vi "OM State Strings 2 Messages.vi"() -> (1 "OM State Strings":T1, 3 "Messages":string)   [LabVIEW 2009]
uses:
  OM State Strings.ctl
  App Status Actions.ctl
  Data Access Objects/Metadata/Persistant DAO Actions.ctl
  Lbcb Control Loop States.ctl
  Data Access Objects/Application/Number Of LBCBs.ctl
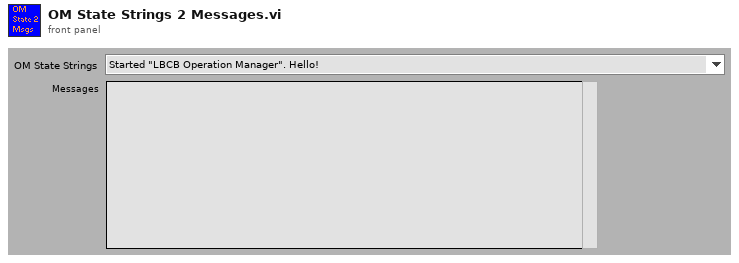
[diagram p1: front panel]
types:
  T1 = typedef "OM State Strings.ctl" = enum16{"Started \"LBCB Operation Manager\". Hello!", "Loading Configuration...", "Setting Up Archiving ...", "Setting Up DAQ Channels...", "Starting Data Acquisition....", "Examine Command from last run ...", "Running  Auto-Balance feedback control loop for LBCB 1 ...", "Running  Auto-Balance feedback control loop for LBCB 2 ...", "Ready to start \"Control\" process for LBCB 1. Push \"Control\" button. ", "Ready to start \"Control\" process for LBCB 2. Push \"Control\" button. ", "LBCB 1 under control", "LBCB 2 under control", "Starting control process. Ready to turn on the pump!", "Stopped \"LBCB Operation Manager\". Bye!"}
  T2 = typedef "Number Of LBCBs.ctl" = enum16{"1", "2"}
  T3 = typedef "Lbcb Control Loop States.ctl" = enum16{"Idle", "Load Last Command", "Start Autobalancing", "Autobalancing", "Control Loop Initialized", "Control Enabled"}
  T4 = typedef "Persistant DAO Actions.ctl" = enum16{"Init", "Get", "Set", "Load", "Save"}
  T5 = typedef "App Status Actions.ctl" = enum16{"Init", "Get Status", "Running", "Control", "Autobalanced", "Data Acquisition", "Set App State", "DAQ Started", "Set LBCB State", "Set All", "Set Cont Logging", "Set Step Logging", "Set MM Logging", "Set Volt Logging", "Set Cart Type", "Set DAQ Link"}
  T6 = typedef "App Status.ctl" = cluster{"Running":bool, "Controlling L2":bool, "Autobalance L2":bool, "Data Acquisition":bool, " App State":T7, "DAQ Started":bool, "LBCB 1 State":T3, "LBCB 2 State":T3, "Controlling L1":bool, "Autobalance L1":bool, "Cartesian Type":bool, "Continuous Logging":bool, "Step Logging":bool, "Voltage Logging":bool, "Mixed Mode Logging":bool, "DAQ Link":bool}
  T7 = typedef "AppStates.ctl" = enum16{"Starting OM", "Initializing Displays", "Setting up Archiving", "Setting Up DAQ Channels", "Start DAQ", "DAQ Starting", "Controlling LBCBs", "Stopping OM"}
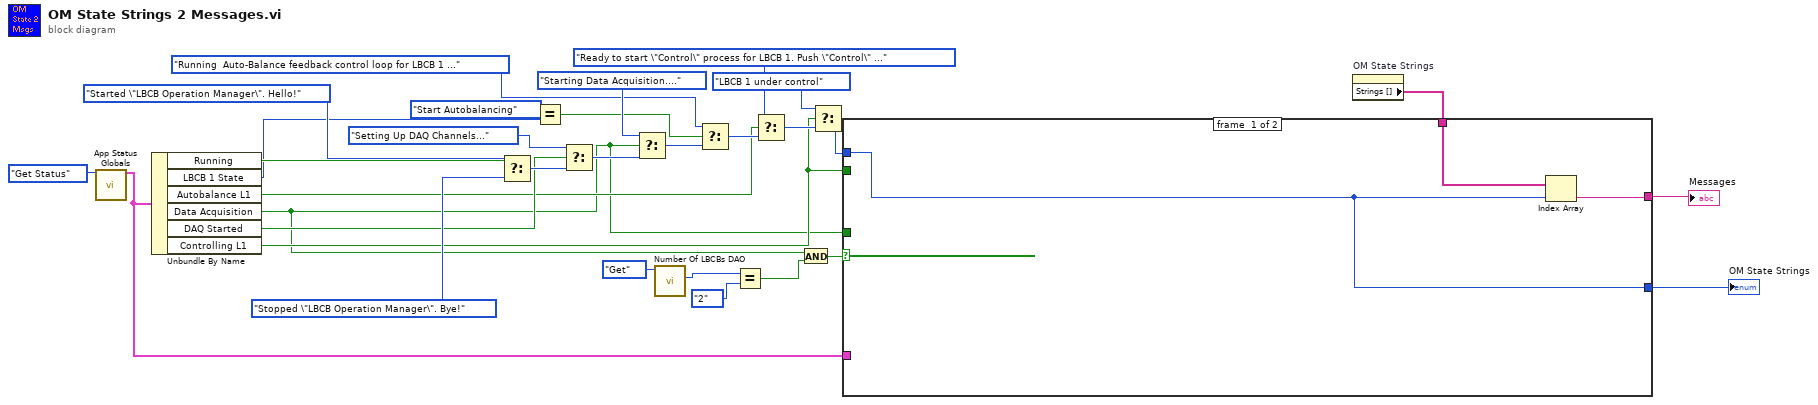
[diagram p0: block diagram]
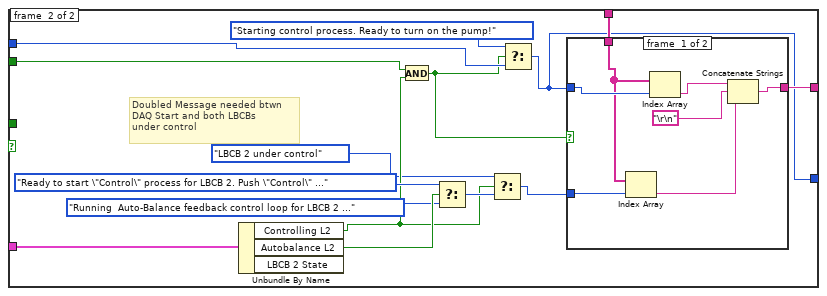
[diagram p2: hidden frame]
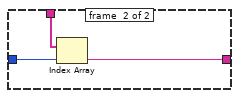
[diagram p3: hidden frame]
diagram:
  n1 = call "App Status Globals.vi"("App Status Actions"=App_Status_Actions."Get Status") -> ("App Status Out"=w11:T6)  [unwired: 5 in, 9 out]
  n2 = Unbundle By Name(w11) -> ("Running"=w31:bool, "LBCB 1 State"=w17:T3, "Autobalance L1"=w4:bool, "Data Acquisition"=w2:bool, "DAQ Started"=w25:bool, "Controlling L1"=w3:bool)
  n3 = Select(t=OM_State_Strings."Started \"LBCB Operation Manager\". Hello!" ("OM State Strings"), s=w31, f=OM_State_Strings."Stopped \"LBCB Operation Manager\". Bye!") -> (s? t:f=w26:T1)
  n4 = Equal?(x=Lbcb_Control_Loop_States."Start Autobalancing", y=w17) -> (x = y?=w5:bool)
  n5 = Select(t=OM_State_Strings."Setting Up DAQ Channels...", s=w25, f=w26) -> (s? t:f=w23:T1)
  n6 = Select(t=OM_State_Strings."Starting Data Acquisition....", s=w2, f=w23) -> (s? t:f=w21:T1)
  n7 = call "Number Of LBCBs DAO.vi"("Actions"=Persistant_DAO_Actions."Get") -> ("Number of\nLBCBs Out"=w15:T2)  [unwired: 3 in, 7 out]
  n8 = Select(t=OM_State_Strings."Running  Auto-Balance feedback control loop for LBCB 1 ...", s=w5, f=w21) -> (s? t:f=w19:T1)
  n9 = Equal?(x=w15, y=Number_Of_LBCBs."2") -> (x = y?=w12:bool)
  n10 = Select(t=OM_State_Strings."Ready to start \"Control\" process for LBCB 1. Push \"Control\" button. ", s=w4, f=w19) -> (s? t:f=w10:T1)
  n11 = And(x=w2, y=w12) -> (x .and. y?=w13:bool)
  n12 = Select(t=OM_State_Strings."LBCB 1 under control", s=w3, f=w10) -> (s? t:f=w8:T1)
  n13 = property on="OM State Strings" class="Enum (strict)"() -> ("Strings []"=w7:string[])  [unwired: 2 in, 2 out]
  n14 = case shown="True" w13 {
    tunnel: w11 -> [_ w49]
    tunnel: w8 -> [w32 w47]
    tunnel: w3 -> [_ w48]
    tunnel: w7 -> [w34 w45]
    tunnel: [w33 w44] -> w6
    tunnel: w2 -> [_ _]
    tunnel: [w32 w35] -> w1
    frame #0 {
      n15 = Index Array(array=w34, index=w32) -> (element=w33:string)
    }
    frame #1 {
      # "Doubled Message needed btwn\nDAQ Start and both LBCBs\nunder control"
      n16 = Unbundle By Name(w49) -> ("Controlling L2"=w38:bool, "Autobalance L2"=w42:bool)  [unwired: 1 out]
      n17 = And(x=w48, y=w38) -> (x .and. y?=w43:bool)
      n18 = Select(t=OM_State_Strings."Ready to start \"Control\" process for LBCB 2. Push \"Control\" button. ", s=w42, f=OM_State_Strings."Running  Auto-Balance feedback control loop for LBCB 2 ...") -> (s? t:f=w39:T1)
      n19 = Select(t=OM_State_Strings."LBCB 2 under control", s=w38, f=w39) -> (s? t:f=w36:T1)
      n20 = Select(t=OM_State_Strings."Starting control process. Ready to turn on the pump!", s=w43, f=w47) -> (s? t:f=w35:T1)
      n21 = case shown="False" w43 {
        tunnel: w45 -> [w55 w59]
        tunnel: w35 -> [w56 w58]
        tunnel: [w53 w57] -> w44
        tunnel: w36 -> [w54 _]
        frame #0 {
          n22 = Index Array(array=w55, index=w54) -> (element=w50:string)
          n23 = Index Array(array=w55, index=w56) -> (element=w52:string)
          n24 = Concatenate Strings(w52, "\r\n", w50) -> (w53:string)
        }
        frame #1 {
          n25 = Index Array(array=w59, index=w58) -> (element=w57:string)
        }
      }
    }
  }
  "OM State Strings" <- w1
  "Messages" <- w6
